vi "Get HS Speed.vi"(7 "speed":sgl, 9 "index":i32, 10 "typ":i32, 11 "channel":i32) -> (3 "function return":u32, 5 "speed out":sgl)   [LabVIEW 2018, in "AndorSDK.lvlib"]
doc: "EXPNETTYPE unsigned int WINAPI GetHSSpeed(int channel, int typ, int index, float * speed);"
uses:
  AndorSDK.lvlib
  ATMCD32D.dll
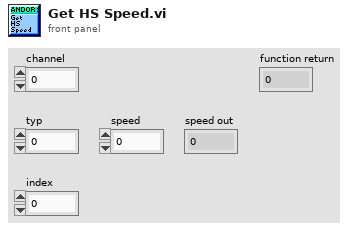
[diagram p1: front panel]
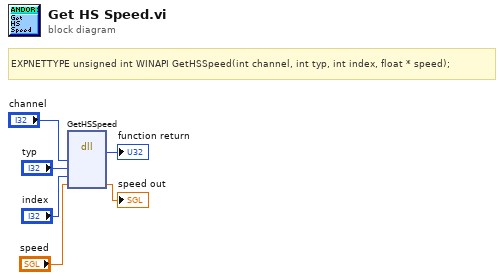
[diagram p0: block diagram]
diagram:
  # "EXPNETTYPE unsigned int WINAPI GetHSSpeed(int channel, int typ, int index, float * speed);"
  n1 = dll-call lib="PTH2babs E\nPersönliches02 - Arbeit03-HiwijobsLabviewCodelibANDOR\tAndor SDK\nATMCD32D.*" fn="GetHSSpeed"("channel"="channel", "typ"="typ", "index"="index", "speed"="speed") -> (→"function return":u32, "speed"=→"speed out":sgl)  [unwired: 6 in, 2 out]
